vi "Example 02a - Basic Lua Scripts.vi"() -> ()   [LabVIEW 2020]
uses:
  Lua for LabVIEW/Lua/Lua.lvclass
panel:
  out "Ё [Number]":dbl[](array[numeric])
  out "Ё [I64]":i64[](array[numeric])
  out "Ё [Boolean]":bool[](array[boolean])
  out "Ё [String]":string[](array[string])
  out "my_number":dbl
  out "my_int":i64
  out "my_bool":bool
  out "my_string":string
  out "error out":errorcluster
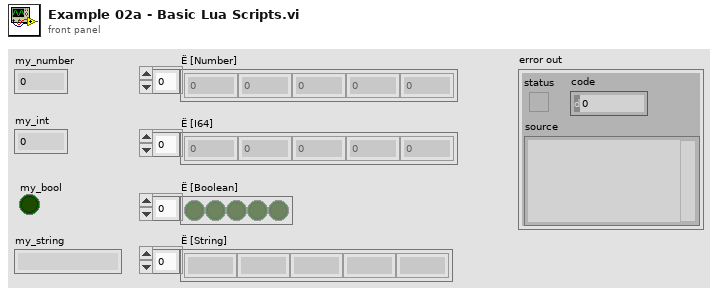
[diagram p1: front panel]
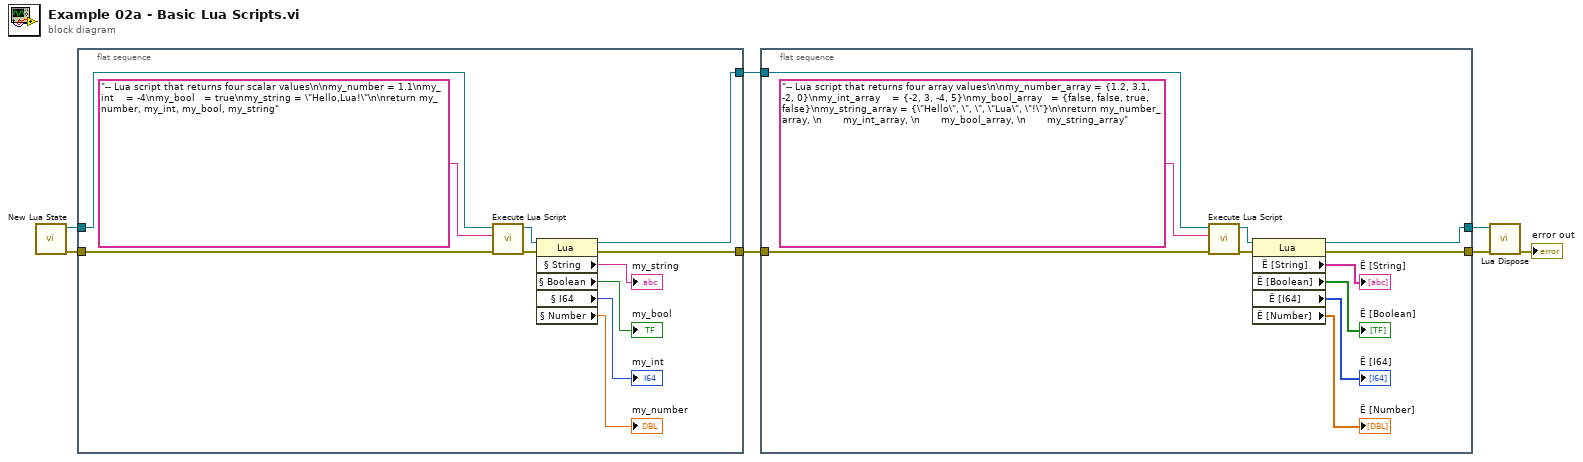
[diagram p0: block diagram]
diagram:
  n1 = call "New Lua State.vi"() -> ("error out"=w6:errorcluster, "Lua out"=w7:refnum<data-value>)  [unwired: 10 in]
  n2 = flat-sequence {
    tunnel: w7 -> [w18]
    tunnel: w6 -> [w16]
    tunnel: [w9] -> w2
    tunnel: [w8] -> w1
    frame #0 {
      n3 = call "Execute Lua Script.vi"("error in (no error)"=w16, "lua script"="-- Lua script that returns four scalar values\n\nmy_number = 1.1\nmy_int    = -4\nmy_bool   = true\nmy_string = \"Hello,Lua!\"\n\nreturn my_number, my_int, my_bool, my_string", "Lua in"=w18) -> ("error out"=w15:errorcluster, "Lua out"=w10:refnum<data-value>)  [unwired: 7 in]
      n4 = property class="Lua"(reference=w10, error in=w15) -> (reference out=w8:refnum<data-value>, error out=w9:errorcluster, "§ String"=→"my_string":string, "§ Boolean"=→"my_bool":bool, "§ I64"=→"my_int":i64, "§ Number"=→"my_number":dbl)
    }
  }
  n5 = flat-sequence {
    tunnel: [w29] -> w4
    tunnel: [w28] -> w3
    tunnel: w2 -> [w23]
    tunnel: w1 -> [w19]
    frame #0 {
      n6 = call "Execute Lua Script.vi"("error in (no error)"=w23, "lua script"="-- Lua script that returns four array values\n\nmy_number_array = {1.2, 3.1, -2, 0}\nmy_int_array    = {-2, 3, -4, 5}\nmy_bool_array   = {false, false, true, false}\nmy_string_array = {\"Hello\", \", \", \"Lua\", \"!\"}\n\nreturn my_number_array, \n       my_int_array, \n       my_bool_array, \n       my_string_array", "Lua in"=w19) -> ("error out"=w21:errorcluster, "Lua out"=w22:refnum<data-value>)  [unwired: 7 in]
      n7 = property class="Lua"(reference=w22, error in=w21) -> (reference out=w29:refnum<data-value>, error out=w28:errorcluster, "Ё [String]"=→"Ё [String]":string[], "Ё [Boolean]"=→"Ё [Boolean]":bool[], "Ё [I64]"=→"Ё [I64]":i64[], "Ё [Number]"=→"Ё [Number]":dbl[])
    }
  }
  n8 = call "Lua Dispose.vi"("error in (no error)"=w3, "Disposable in"=w4) -> ("error out"=→"error out":errorcluster)  [unwired: 9 in]
